vi "Done Reading File.vi"(6 "gain":dbl, 7 "dt":dbl, 8 "error in (no error)":errorcluster, 9 "Read Speed":dbl, 10 "Data Buffer":T1, 11 "TDMS Data Source in":refnum<class "TDMS Data Source.lvclass">) -> (0 "error out":errorcluster, 3 "TDMS Data Source out":refnum<class "TDMS Data Source.lvclass">)   [LabVIEW 2020, in "TDMS Data Source.lvlib" / "TDMS Data Source.lvclass"]
uses:
  TDMS Data Source.lvclass
  C:/Program Files/National Instruments/LabVIEW 2026/vi.lib/ActorFramework/Actor/Actor.lvclass
  GPU FFT Calculator/GPU FFT Calculator/Data Source Buffer.ctl
  <vilib>/ActorFramework/Actor/Actor.lvclass/Actor.ctl
  TDMS Data Source.lvclass/TDMS Data Source.ctl
  <vilib>/ActorFramework/Message Enqueuer/Message Enqueuer.lvclass/Message Enqueuer.ctl
  Data Source/Data Source Messages/Continue Acquisition Msg/Continue Acquisition Msg.lvclass/Continue Acquisition Msg.ctl
  Application Manager/Application Manager Messages/Update Data Buffer Msg/Update Data Buffer Msg.lvclass/Update Data Buffer Msg.ctl
  Application Manager/Application Manager Messages/Update Data Source Read Speed Msg/Update Data Source Read Speed Msg.lvclass/Update Data Source Read Speed Msg.ctl
  <vilib>/ActorFramework/Message Enqueuer/Init from Existing Queue.vi
  <vilib>/ActorFramework/Message Enqueuer/Enqueue.vi
  Data Source/Data Source Messages/Continue Acquisition Msg/Continue Acquisition Msg.lvclass
  C:/Program Files/National Instruments/LabVIEW 2026/vi.lib/ActorFramework/Message/Message.lvclass
  Application Manager/Application Manager Messages/Update Data Buffer Msg/Update Data Buffer Msg.lvclass
  Application Manager/Application Manager Messages/Update Data Source Read Speed Msg/Update Data Source Read Speed Msg.lvclass
  <vilib>/ActorFramework/Message Priority Queue/Priority Enqueue.vi
  <vilib>/ActorFramework/Message Enqueuer/Message Enqueuer.lvclass
  <vilib>/ActorFramework/Actor/Actor.lvclass
  Data Source/Data Source/Data Source.lvclass
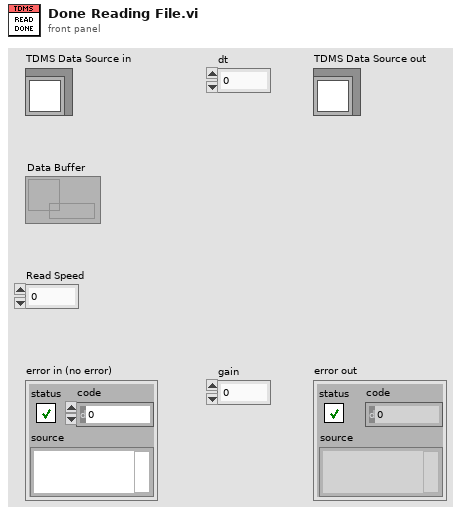
[diagram p1: front panel]
types:
  T1 = typedef "Data Source.lvlib/Data Source.lvclass/Data Source Buffer.ctl" = refnum<data-value>
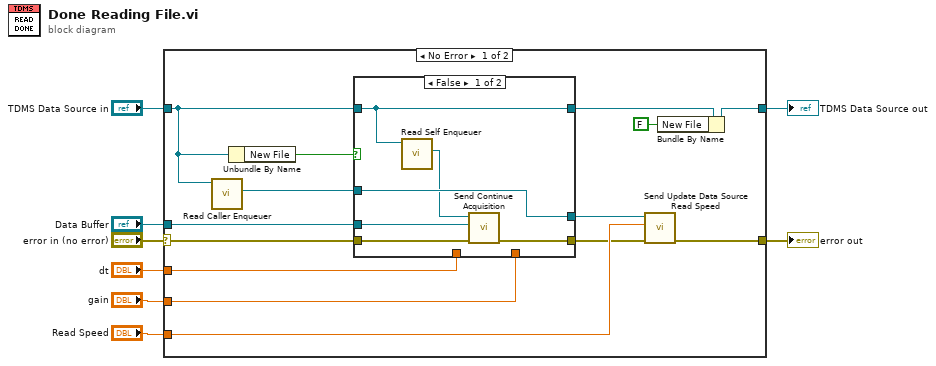
[diagram p0: block diagram]
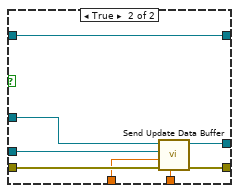
[diagram p2: hidden frame]
diagram:
  n1 = case shown="No Error" "error in (no error)" {
    selector: "error in (no error)" -> [w16 w38]
    tunnel: [w21 w38] -> w7
    tunnel: [w12 w37] -> w5
    tunnel: "TDMS Data Source in" -> [w13 w37]
    tunnel: "Data Buffer" -> [w17 _]
    tunnel: "Read Speed" -> [w22 _]
    tunnel: "dt" -> [w10 _]
    tunnel: "gain" -> [w9 _]
    frame No Error {
      n2 = call <vilib>:"Read Caller Enqueuer.vi"("Actor"=w13) -> ("Caller Enqueuer"=w20:refnum<class "Message Enqueuer.lvclass">)  [unwired: 10 in]
      n3 = Unbundle By Name(w13) -> ("New File"=w15:bool)
      n4 = case shown="False" w15 {
        tunnel: w20 -> [w28 w36]
        tunnel: [w28 w35] -> w19
        tunnel: [w23 w34] -> w18
        tunnel: w17 -> [w25 w33]
        tunnel: w16 -> [w24 w32]
        tunnel: [w27 w31] -> w14
        tunnel: w13 -> [w27 w31]
        tunnel: w10 -> [_ w30]
        tunnel: w9 -> [_ w29]
        frame False {
          n5 = call <vilib>:"Read Self Enqueuer.vi"("Actor"=w27) -> ("Self Enqueuer"=w26:refnum<class "Message Enqueuer.lvclass">)  [unwired: 10 in]
          n6 = call "Send Continue Acquisition.vi"("error in (no error)"=w24, "Data Buffer"=w25, "Message Enqueuer"=w26) -> ("error out"=w23:errorcluster)  [unwired: 7 in, 1 out]
        }
        frame True {
          n7 = call "Send Update Data Buffer.vi"("gain"=w29, "error in (no error)"=w32, "dt"=w30, "Data Buffer"=w33, "Message Enqueuer"=w36) -> ("error out"=w34:errorcluster, "Message Enqueuer out"=w35:refnum<class "Message Enqueuer.lvclass">)  [unwired: 5 in]
        }
      }
      n8 = call "Send Update Data Source Read Speed.vi"("error in (no error)"=w18, "Read Speed (GB/s)"=w22, "Message Enqueuer"=w19) -> ("error out"=w21:errorcluster)  [unwired: 7 in, 1 out]
      n9 = Bundle By Name(cluster=w14, "New File"=FALSE) -> (w12:refnum<class "TDMS Data Source.lvclass">)
    }
    frame Error {
    }
  }
  "error out" <- w7
  "TDMS Data Source out" <- w5
